vi "UDP Test for CAN0.vi"() -> ()   [LabVIEW 2015]
uses:
  <vilib>/FPGAPlugInAG/cRIO-9063/niLvFpga_Open_cRIO-9063.vi
  <vilib>/rvi/interface/common/dynamic/niFpgaDynamicAddResources.vi
  <vilib>/Utility/error.llb/Error Cluster From Error Code.vi
  <vilib>/rvi/errors/niLvFpgaAdjustHostInterfaceError.vi
  <vilib>/FPGAPlugInAG/Dynamic/niLvFpga_Close_Dynamic.vi
  <vilib>/rvi/interface/nirviOpenFPGA/nirviOpenFPGA.xnode
  FPGA Bitfiles/VCU-VEHICLEMODEL_FPGATarget_CANBasic(FPGA)_WVt1gIpoBPw.lvbitx
  Basic (FPGA) CAN Engine .vi
  <vilib>/rvi/interface/nirviReadWriteControl/nirviReadWriteControl.xnode
  <vilib>/rvi/interface/nirviCloseFPGA/nirviCloseFPGA.xnode
  <vilib>/rvi/interface/Simulation/niFpgaSimulationCallBeginRW.vi
  NiFpgaLv.dll
panel:
  in  "Start":bool
  out "Loop time":sgl
  out "Old Timestamp":u64
  out "No# Frames Sent":i32
  out "error out":errorcluster
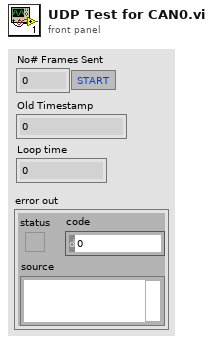
[diagram p1: front panel]
types:
  T1 = enum8{"Data Frame", "Remote Frame", "(reserved)", "(reserved) ", "(reserved)  ", "(reserved)   ", "Bus Error", "Transceiver Fault"}
  T2 = cluster{u32, u32, u32, "type":enum8{"Data Frame", "Remote Frame", "(reserved)", "(reserved) ", "(reserved)  ", "(reserved)   ", "Bus Error", "Transceiver Fault"}, u8, u8, u8, u8[]}
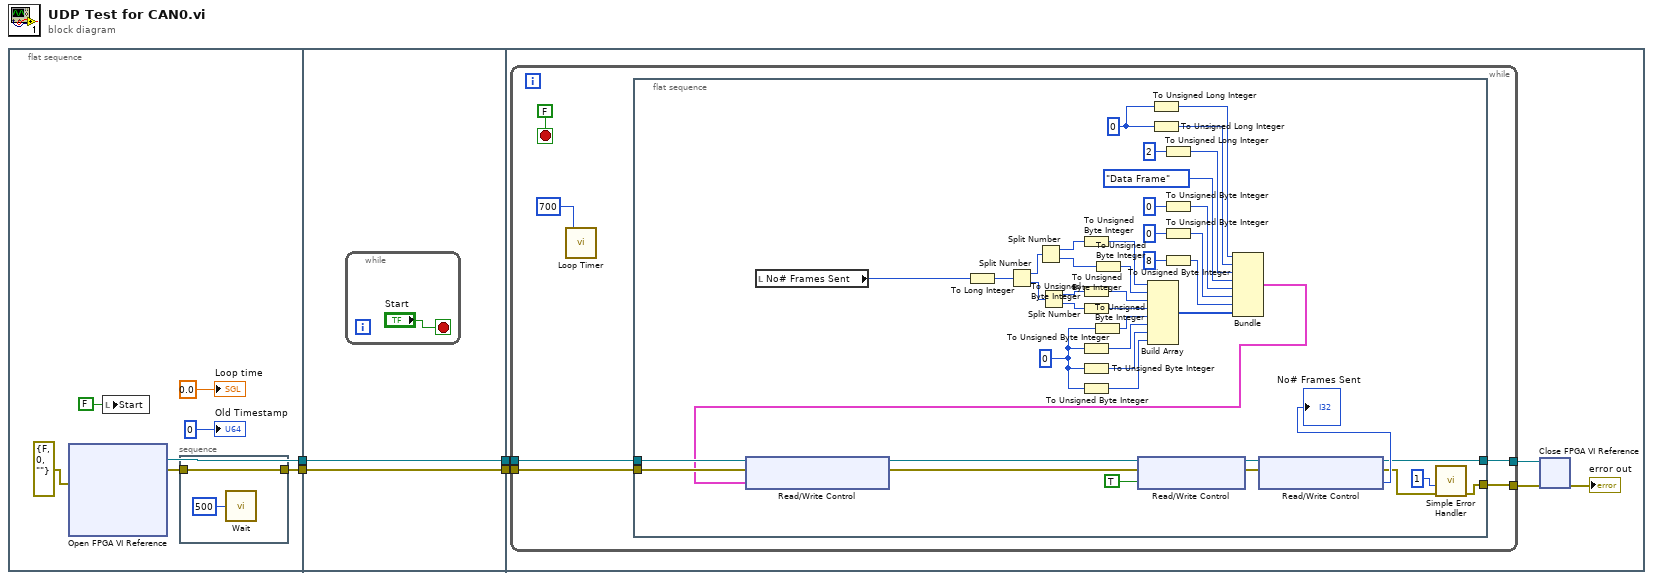
[diagram p0: block diagram]
diagram:
  n1 = flat-sequence {
    tunnel: [w9] -> w4
    tunnel: [w8] -> w2
    tunnel: w4 -> [w15]
    tunnel: [w15] -> w3
    tunnel: w2 -> [w14]
    tunnel: [w14] -> w1
    tunnel: w3 -> [w18]
    tunnel: w1 -> [w17]
    frame #0 {
      n2 = xnode "Open FPGA VI Reference"("error in"=errorcluster {"status"=FALSE, "code"=0, "source"=""}) -> ("FPGA VI Reference Out"=w8:refnum<k20>, "error out"=w10:errorcluster)  [unwired: 1 in]
      n3 = local write "Start"(FALSE ("Start")) -> ()
      n4 = stacked-sequence {
        tunnel: w10 -> [w13]
        tunnel: [w13] -> w9
        frame #0 {
          n5 = call "Wait"("Count(mSec)"=u32 500) -> ()  [unwired: 1 out]
        }
      }
      "Loop time" <- sgl 0.0 ("Loop time")
      "Old Timestamp" <- u64 0 ("Old Timestamp")
    }
    frame #1 {
      n6 = while {
        stop <- "Start" stop-if-true
      }
    }
    frame #2 {
      n7 = while {
        tunnel: [w26] -> w20
        tunnel: [w25] -> w19
        tunnel: w17 -> [w22]
        tunnel: w18 -> [w23]
        stop <- FALSE stop-if-true
        n8 = call "Loop Timer"("Count(mSec)"=u32 700) -> ()  [unwired: 1 out]
        n9 = flat-sequence {
          tunnel: [w34] -> w26
          tunnel: [w36] -> w25
          tunnel: w22 -> [w38]
          tunnel: w23 -> [w33]
          frame #0 {
            w45 = i16 0
            w69 = i16 0
            n10 = local read "No# Frames Sent"() -> (w28:i32)
            n11 = To Long Integer(number=w28) -> (32bit integer=w49:i32)
            n12 = Split Number(x=w49) -> (hi(x)=w29:u16, lo(x)=w48:u16)
            n13 = Split Number(x=w29) -> (hi(x)=w30:u8, lo(x)=w31:u8)
            n14 = Split Number(x=w48) -> (hi(x)=w47:u8, lo(x)=w46:u8)
            n15 = To Unsigned Byte Integer(number=w30) -> (unsigned 8bit integer=w59:u8)
            n16 = To Unsigned Byte Integer(number=w47) -> (unsigned 8bit integer=w57:u8)
            n17 = To Unsigned Byte Integer(number=w46) -> (unsigned 8bit integer=w56:u8)
            n18 = To Unsigned Byte Integer(number=w45) -> (unsigned 8bit integer=w54:u8)
            n19 = To Unsigned Byte Integer(number=w45) -> (unsigned 8bit integer=w53:u8)
            n20 = To Unsigned Byte Integer(number=w45) -> (unsigned 8bit integer=w52:u8)
            n21 = To Unsigned Byte Integer(number=w45) -> (unsigned 8bit integer=w55:u8)
            n22 = To Unsigned Byte Integer(number=w31) -> (unsigned 8bit integer=w58:u8)
            n23 = Build Array(w59, w58, w57, w56, w55, w54, w53, w52) -> (w50:u8[])
            n24 = To Unsigned Long Integer(number=w69) -> (unsigned 32bit integer=w65:u32)
            n25 = To Unsigned Long Integer(number=w69) -> (unsigned 32bit integer=w64:u32)
            n26 = To Unsigned Long Integer(number=i16 2) -> (unsigned 32bit integer=w63:u32)
            n27 = To Unsigned Byte Integer(number=u8 0 ("info A")) -> (unsigned 8bit integer=w62:u8)
            n28 = To Unsigned Byte Integer(number=u8 0 ("info B")) -> (unsigned 8bit integer=w61:u8)
            n29 = To Unsigned Byte Integer(number=i16 8) -> (unsigned 8bit integer=w60:u8)
            n30 = Bundle(w65, w64, w63, "type"=T1."Data Frame", w62, w61, w60, w50) -> (w32:T2)  [unwired: 1 in]
            n31 = xnode "Read/Write Control"("FPGA VI Reference In"=w38, "error in"=w33, "CAN0 - Transmit Frame"=w32) -> ("FPGA VI Reference Out"=w37:refnum<k20>, "error out"=w35:errorcluster)
            n32 = xnode "Read/Write Control"("FPGA VI Reference In"=w37, "error in"=w35, "CAN0 - Transmit"=TRUE) -> ("FPGA VI Reference Out"=w41:refnum<k20>, "error out"=w44:errorcluster)
            n33 = xnode "Read/Write Control"("FPGA VI Reference In"=w41, "error in"=w44) -> ("FPGA VI Reference Out"=w36:refnum<k20>, "error out"=w42:errorcluster, "CAN0 - Frames Sent"=→"No# Frames Sent":u32)
            n34 = call <vilib>:"Simple Error Handler.vi"("type of dialog (OK msg:1)"=1, "error in (no error)"=w42) -> ("error out"=w34:errorcluster)  [unwired: 3 in, 4 out]
          }
        }
      }
      n35 = xnode "Close FPGA VI Reference"("FPGA VI Reference In"=w19, "error in"=w20) -> ("error out"=→"error out":errorcluster)
    }
  }
